vi "Get_Device_Properties.vi"(3 "IP Address":string) -> (1 "Device Properties":string[](array[string]))   [LabVIEW 2024]
uses:
  <vilib>/numeric/Random Number (Range) U64.vi
  <vilib>/numeric/sub_Random U32.vi
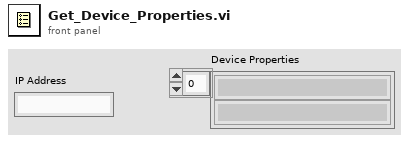
[diagram p1: front panel]
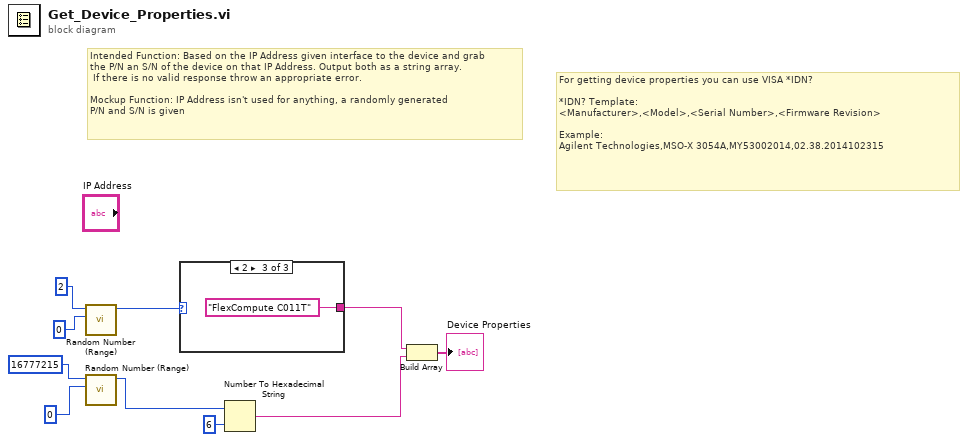
[diagram p0: block diagram]
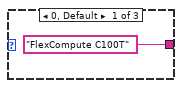
[diagram p2: hidden frame]
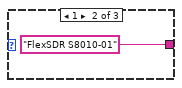
[diagram p3: hidden frame]
diagram:
  # "For getting device properties you can use VISA *IDN?\n\n*IDN? Template:\n<Manufacturer>,<Model>,<Serial Number>,<Firmware Revision>\n\nExample:\nAgilent Technologies,MSO-X 3054A,MY53002014,02.38.2014102315"
  # "Intended Function: Based on the IP Address given interface to the device and grab\nthe P/N an S/N of the device on that IP Address. Output both as a string array.\n If there is no valid response throw an appropriate error.\n\nMockup Function: IP Address isn't used for anything, a randomly generated \nP/N and S/N is given"
  n1 = call-poly <vilib>:"Random Number (Range).vi"("lower bound (0)"=u64 0, "upper bound (100)"=u64 2) -> ("number"=w8:u64)  [unwired: 9 in]
  n2 = call-poly <vilib>:"Random Number (Range).vi"("lower bound (0)"=u64 0, "upper bound (100)"=u64 16777215 ("lower bound (0)")) -> ("number"=w2:u64)  [unwired: 9 in]
  n3 = case shown="2" w8 {
    tunnel: ["FlexCompute C100T" "FlexSDR S8010-01" "FlexCompute C011T"] -> w5
    frame 0, Default {
    }
    frame 1 {
    }
    frame 2 {
    }
  }
  n4 = Number To Hexadecimal String(1:i16 6 ("width (-)"), 2:w2) -> (0:w4:string)
  n5 = Build Array(w5, w4) -> (→"Device Properties":string[])
